vi "data logger_lvm.vi"() -> ()   [LabVIEW 2010]
panel:
  out "2D Array":dbl[][](array[numeric]) format="%.4f"
  in  "# of Columns":u8
  in  "# of Rows":u8
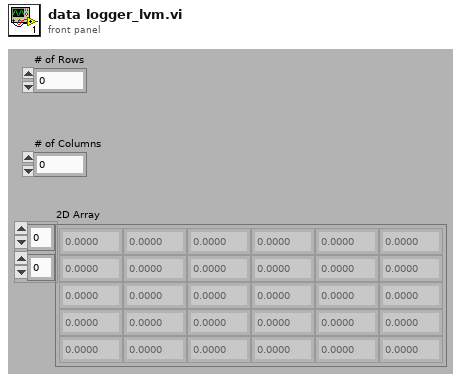
[diagram p1: front panel]
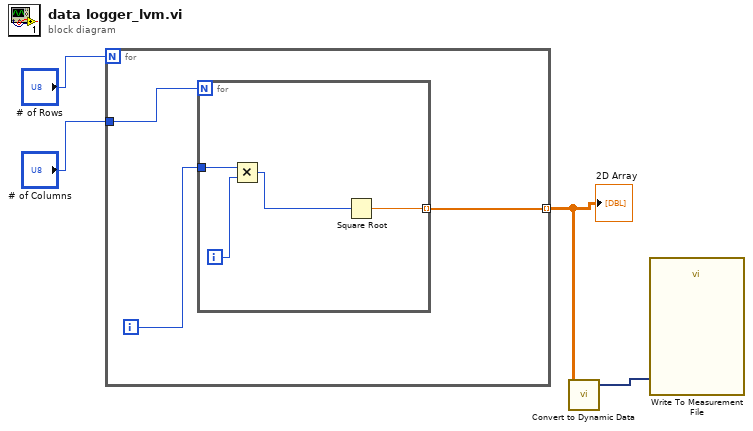
[diagram p0: block diagram]
diagram:
  n1 = for {
    N: "# of Rows" -> [_]
    tunnel: "# of Columns" -> [w6]
    tunnel: [w5] -> w1 mode=indexing
    i -> [w7]
    n2 = for {
      N: w6 -> [_]
      tunnel: w7 -> [w11]
      tunnel: [w8] -> w5 mode=indexing
      i -> [w10]
      n3 = Multiply(x=w11, y=w10) -> (x*y=w9:i32)
      n4 = Square Root(x=w9) -> (sqrt(x)=w8:dbl)
    }
  }
  "2D Array" <- w1
  n5 = call "Convert to Dynamic Data"("2D Array"=w1) -> ("Dynamic Data Type"=w2:dynamicdata)  [unwired: 3 in]
  n6 = call "Write To Measurement File"("Signals"=w2) -> ()  [unwired: 16 in, 3 out]
